vi "LWESP301_Close.vi"(2 "error in (no error)":errorcluster caption="error in", 4 "ESP301 Reference":refnum<k24>) -> (0 "Error out":errorcluster caption="error out")   [LabVIEW 2015]
uses:
  Newport.ESP301.CommandInterface
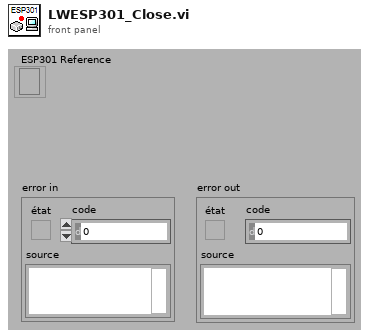
[diagram p1: front panel]
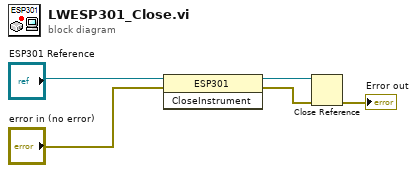
[diagram p0: block diagram]
diagram:
  n1 = invoke class="ESP301" method="CloseInstrument"(reference="ESP301 Reference", error in="error in (no error)") -> (reference out=w5:refnum<k24>, error out=w4:errorcluster)  [unwired: 1 in, 1 out]
  n2 = Close Reference(reference=w5, error in (no error)=w4) -> (error out=→"Error out":errorcluster)
